vi "swabian_logto_dotPhotons.vi"(8 "error in (no error)":errorcluster, 11 "swabian_local_data":T1={"events"={"update_status"=refnum, "update_chart"=refnum, "update_xy"=refnum, "send_channel_data"=refnum}, "stop_q"=refnum, "tagger_reference"=refnum, "connect_button"=refnum, "counter_reference"=refnum, "tagger_stream_reference"=refnum, "log_reference"=refnum, "current_log_offset"=0, "tt20_buffer_q"=refnum, "stream_to_file_button"=refnum, "num_records"=0, "connected?"=FALSE, "plots"=refnum, "histogram_bin_edges"=[], "histogrammer"=refnum, "plot_lifetimes"=refnum, "xy_graph"=refnum, "Reference\nChannel"=enum."ch0", "trigger_channels"=[], "filter_channels"=[], "active_channels"=[], "acq_mode"=0, "Reference\nChannel"=enum."ch0", "acq_time"=0, "leftovers"={"leftover_stamps"=[], "leftover_channels"=[], "any?"=FALSE}, "sync_period_ps"=0, "raw_stream_path"=path "", "Leftovers"={"missing_sync_data"=[], "missing_events"=0}, "first_batch"=0, "first_sync_stamp"=0, "lifetime_settings"={"Plot Lifetimes"=FALSE, "start_time"=0.0, "stop_time"=0.0, "n_bins"=0}, "Histogram_bins"=[], "last_processed_data"=[], "histogram_data"=[]}) -> (0 "error out":errorcluster, 2 "stop_loop":bool, 3 "swabian_local_data 2":T1={"events"={"update_status"=refnum, "update_chart"=refnum, "update_xy"=refnum, "send_channel_data"=refnum}, "stop_q"=refnum, "tagger_reference"=refnum, "connect_button"=refnum, "counter_reference"=refnum, "tagger_stream_reference"=refnum, "log_reference"=refnum, "current_log_offset"=0, "tt20_buffer_q"=refnum, "stream_to_file_button"=refnum, "num_records"=0, "connected?"=FALSE, "plots"=refnum, "histogram_bin_edges"=[], "histogrammer"=refnum, "plot_lifetimes"=refnum, "xy_graph"=refnum, "Reference\nChannel"=enum."ch0", "trigger_channels"=[], "filter_channels"=[], "active_channels"=[], "acq_mode"=0, "Reference\nChannel"=enum."ch0", "acq_time"=0, "leftovers"={"leftover_stamps"=[], "leftover_channels"=[], "any?"=FALSE}, "sync_period_ps"=0, "raw_stream_path"=path "", "Leftovers"={"missing_sync_data"=[], "missing_events"=0}, "first_batch"=0, "first_sync_stamp"=0, "lifetime_settings"={"Plot Lifetimes"=FALSE, "start_time"=0.0, "stop_time"=0.0, "n_bins"=0}, "Histogram_bins"=[], "last_processed_data"=[], "histogram_data"=[]})   [LabVIEW 2018]
uses:
  swabian_local_data_tdef.ctl
  swabian_events_tdef.ctl
  update_chart_tdef.ctl
  channel_data_tdef.ctl
  C:/Users/bspoka/Documents/swabian_LV/lib/TTCSharp32.dll
  lib/TTCSharp32.dll
  swabian_buffer_tdef.ctl
  reference_checkbox_tdef.ctl
  leftovers_struct.ctl
  lifetime_settings.ctl
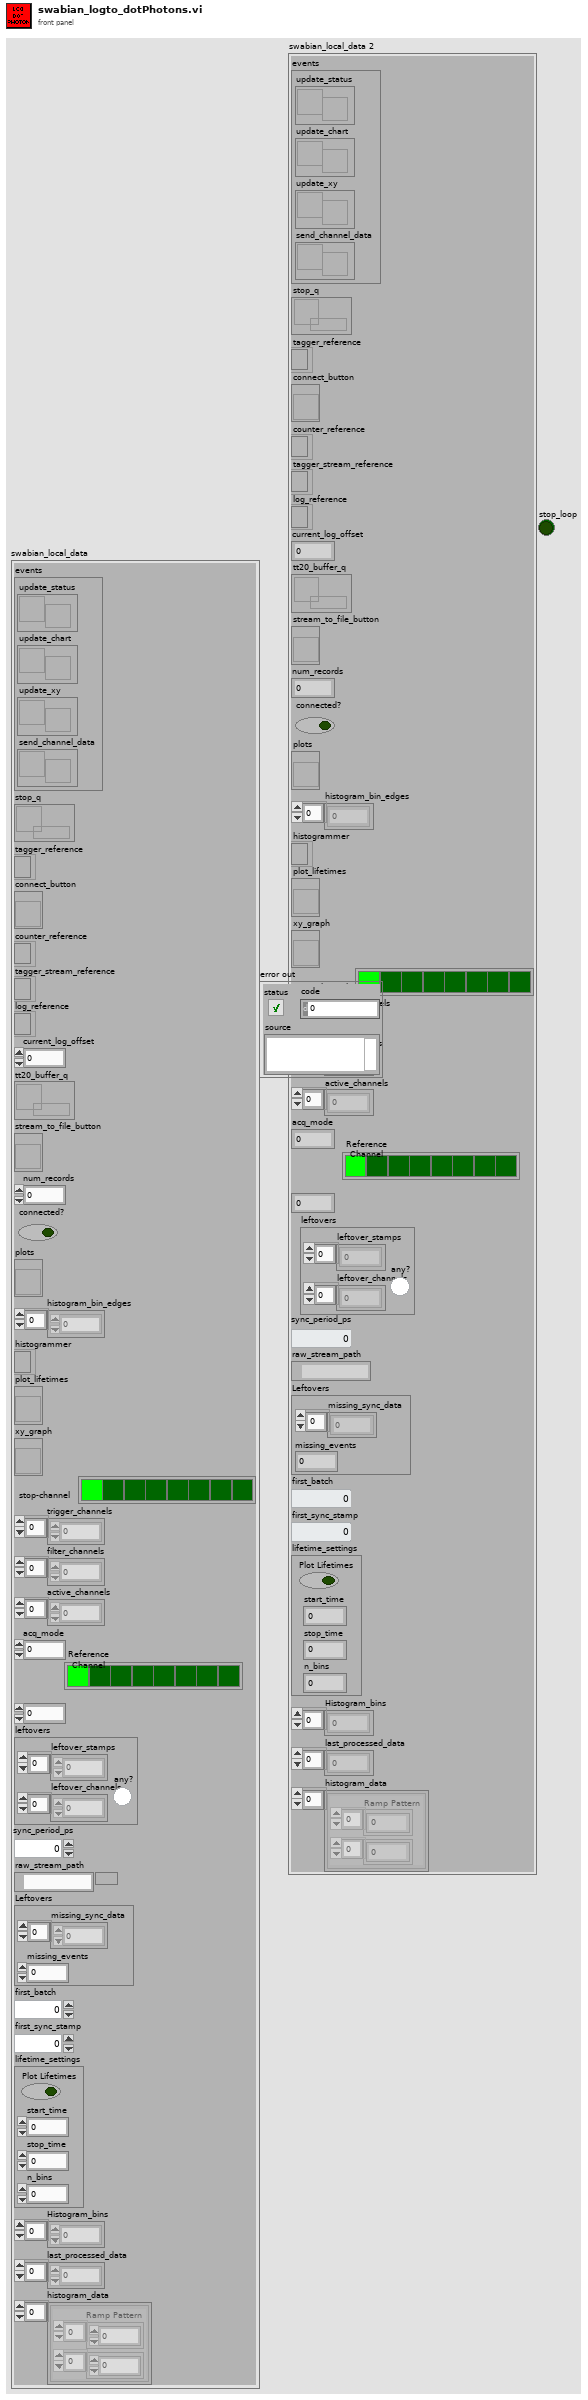
[diagram p1: front panel]
types:
  T1 = typedef "swabian_local_data_tdef.ctl" = cluster{"events":T2, "stop_q":refnum<queue>, "tagger_reference":refnum<k24>, "connect_button":refnum<vi>, "counter_reference":refnum<k24>, "tagger_stream_reference":refnum<k24>, "log_reference":refnum<file>, "current_log_offset":i64, "tt20_buffer_q":refnum<queue>, "stream_to_file_button":refnum<vi>, "num_records":u64, "connected?":bool, "plots":refnum<vi>, "histogram_bin_edges":i64[], "histogrammer":refnum<k24>, "plot_lifetimes":refnum<vi>, "xy_graph":refnum<vi>, "Reference\nChannel":T3, "trigger_channels":i32[], "filter_channels":i32[], "active_channels":i32[], "acq_mode":i32, "Reference\nChannel":T3, "acq_time":i64, "leftovers":T4, "sync_period_ps":i64, "raw_stream_path":path, "Leftovers":cluster{"missing_sync_data":u64[], "missing_events":i32}, "first_batch":i32, "first_sync_stamp":u64, "lifetime_settings":T5, "Histogram_bins":dbl[], "last_processed_data":u64[], "histogram_data":cluster{"Ramp Pattern":dbl[], dbl[]}[]}
  T2 = typedef "swabian_events_tdef.ctl" = cluster{"update_status":refnum<user-event>, "update_chart":refnum<user-event>, "update_xy":refnum<user-event>, "send_channel_data":refnum<user-event>}
  T3 = typedef "reference_checkbox_tdef.ctl" = enum32{"No Selection", "ch0", "ch1", "ch2", "ch3", "ch4", "ch5", "ch6", "ch7"}
  T4 = typedef "leftovers_struct.ctl" = cluster{"leftover_stamps":i64[], "leftover_channels":i32[], "any?":bool}
  T5 = typedef "lifetime_settings.ctl" = cluster{"Plot Lifetimes":bool, "start_time":dbl, "stop_time":dbl, "n_bins":i32}
  T6 = enum16{"big-endian, network order", "native, host order", "little-endian"}
  T7 = cluster{"missing_sync_data":u64[], "missing_events":i32}
  T8 = typedef "swabian_buffer_tdef.ctl" = cluster{"tagChannels":i32[], "tagTimestamps":i64[], "size":i32}
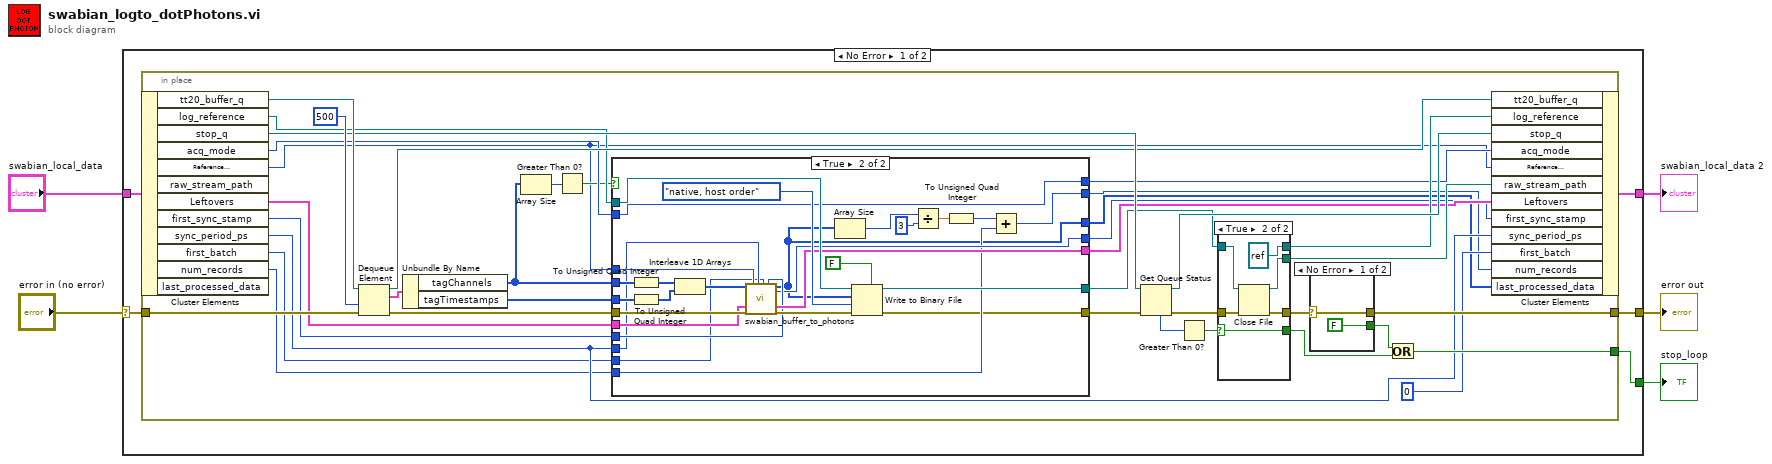
[diagram p0: block diagram]
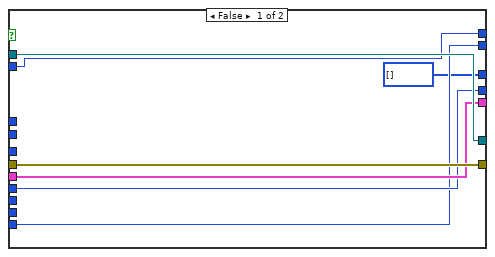
[diagram p2: hidden frame]
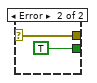
[diagram p3: hidden frame]
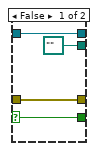
[diagram p4: hidden frame]
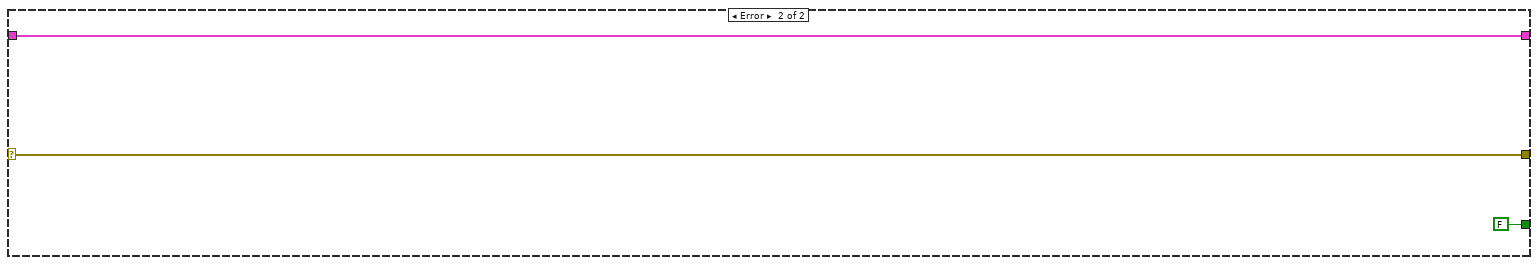
[diagram p5: hidden frame]
diagram:
  n1 = case shown="No Error" "error in (no error)" {
    selector: "error in (no error)" -> [w9 w98]
    tunnel: "swabian_local_data" -> [w10 w97]
    tunnel: [w7 w98] -> w1
    tunnel: [w8 w97] -> w3
    tunnel: [w6 FALSE] -> w2
    frame No Error {
      n2 = in-place {
        in-place-border: w9 -> [w46]
        in-place-border: [w32] -> w7
        in-place-border: [w34] -> w6
        n3 = in-place-cluster #1(w10) -> ("tt20_buffer_q"=w48:refnum<queue>, "log_reference"=w30:refnum<file>, "stop_q"=w43:refnum<queue>, "acq_mode"=w28:i32, "Reference\nChannel"=w22:T3, "Leftovers"=w20:T7, "first_sync_stamp"=w18:u64, "sync_period_ps"=w16:i64, "first_batch"=w15:i32, "num_records"=w13:u64)  [unwired: 2 out]
        n4 = Dequeue Element(queue=w48, timeout in ms (-1)=500, error in (no error)=w46) -> (queue out=w31:refnum<queue>, element=w45:T8, error out=w29:errorcluster)  [unwired: 1 out]
        n5 = Unbundle By Name(w45) -> ("tagChannels"=w24:i32[], "tagTimestamps"=w23:i64[])
        n6 = Array Size(array=w24) -> (size(s)=w26:i32)
        n7 = Greater Than 0?(x=w26) -> (x > 0?=w25:bool)
        n8 = case shown="True" w25 {
          tunnel: [w55 w57] -> w44
          tunnel: [w54 w81] -> w39
          tunnel: w30 -> [w54 w80]
          tunnel: w29 -> [w55 w72]
          tunnel: w28 -> [w53 w76]
          tunnel: w23 -> [_ w78]
          tunnel: w24 -> [_ w77]
          tunnel: [w53 w76] -> w27
          tunnel: w22 -> [_ w66]
          tunnel: w20 -> [w52 w70]
          tunnel: [w52 w69] -> w19
          tunnel: w18 -> [w51 w68]
          tunnel: [w51 w67] -> w17
          tunnel: w16 -> [_ w65]
          tunnel: w15 -> [_ w64]
          tunnel: w13 -> [w50 w61]
          tunnel: [w50 w58] -> w12
          tunnel: [u64[] [] ("output_buffer") w56] -> w11
          frame False {
          }
          frame True {
            n9 = To Unsigned Quad Integer(1:w77) -> (0:w75:u64[])
            n10 = To Unsigned Quad Integer(1:w78) -> (0:w74:u64[])
            n11 = Interleave 1D Arrays(w75, w74) -> (w73:u64[])
            n12 = call "swabian_buffer_to_photons.vi"("buffer"=w73, "Leftovers_in"=w70, "error in (no error)"=w72, "sync_channel"=w66, "sync_period_ps"=w65, "first_batch"=w64, "first_sync_stamp"=w68) -> ("output_buffer"=w56:u64[], "first_sync_stamp_out"=w67:u64, "Leftovers_out"=w69:T7, "error out"=w71:errorcluster)  [unwired: 9 in]
            n13 = Array Size(array=w56) -> (size(s)=w63:i32)
            n14 = Write to Binary File(file (use dialog)=w80, data=w56, error in=w71, 5:FALSE ("prepend array or string size? (T)"), 9:T6."native, host order" ("byte order (0:big-endian, network order)")) -> (refnum out=w81:refnum<file>, error out=w57:errorcluster)  [unwired: 1 in, 1 out]
            n15 = Divide(x=w63, y=3) -> (x/y=w60:dbl)
            n16 = To Unsigned Quad Integer(1:w60) -> (0:w59:u64)
            n17 = Add(x=w59, y=w61) -> (x+y=w58:u64)
          }
        }
        n18 = Get Queue Status(queue=w43, error in (no error)=w44) -> (queue out=w42:refnum<queue>, error out=w38:errorcluster, # elements in queue=w41:i32)  [unwired: 1 in, 5 out]
        n19 = Greater Than 0?(x=w41) -> (x > 0?=w40:bool)
        n20 = case shown="True" w40 {
          selector: w40 -> [w89 w92]
          tunnel: w39 -> [w90 w96]
          tunnel: w38 -> [w88 w95]
          tunnel: [w90 refnum<file> refnum ("refnum out")] -> w37
          tunnel: [w88 w93] -> w36
          tunnel: [w89 w92] -> w33
          tunnel: [path "" ("path") w91] -> w21
          frame False {
          }
          frame True {
            n21 = Close File(refnum=w96, error in=w95) -> (path=w91:path, error out=w93:errorcluster)
          }
        }
        n22 = case shown="No Error" w36 {
          selector: w36 -> [w83 w85]
          tunnel: [FALSE TRUE] -> w35
          tunnel: [w83 w85] -> w32
          frame No Error {
          }
          frame Error {
          }
        }
        n23 = Or(x=w35, y=w33) -> (x .or. y?=w34:bool)
        n24 = in-place-cluster #1("tt20_buffer_q"=w31, "log_reference"=w37, "stop_q"=w42, "acq_mode"=w27, "Reference\nChannel"=w22, "raw_stream_path"=w21, "Leftovers"=w19, "first_sync_stamp"=w17, "sync_period_ps"=w16, "first_batch"=0, "num_records"=w12, "last_processed_data"=w11) -> (w8:T1)
      }
    }
    frame Error {
    }
  }
  "swabian_local_data 2" <- w3
  "error out" <- w1
  "stop_loop" <- w2
